vi "ZoomAndCenterImage.vi"(8 "error in (no error)":errorcluster, 10 "image data":T1, 11 "Picture Ref":refnum<vi>) -> (0 "error out":errorcluster)   [LabVIEW 2015]
uses:
  <vilib>/picture/picture.llb/imagedata.ctl
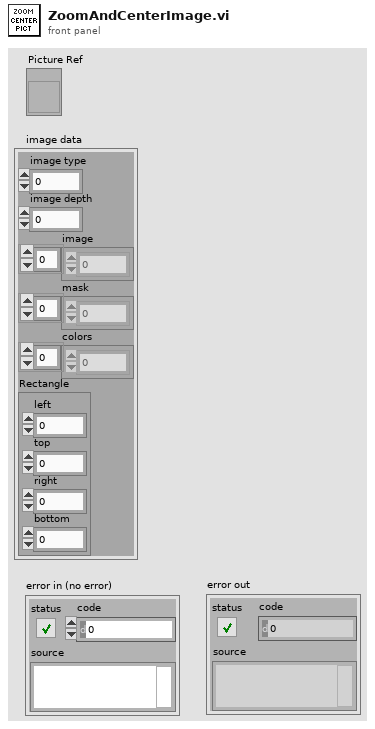
[diagram p1: front panel]
types:
  T1 = typedef "imagedata.ctl" = cluster{"image type":i32, "image depth":i32, "image":u8[], "mask":u8[], "colors":u32[], "Rectangle":cluster{"left":i16, "top":i16, "right":i16, "bottom":i16}}
  T2 = cluster{"left":i16, "top":i16, "right":i16, "bottom":i16}
  T3 = typedef "LVBoundsTypeDef.ctl" = cluster{"Width":u32, "Height":u32}
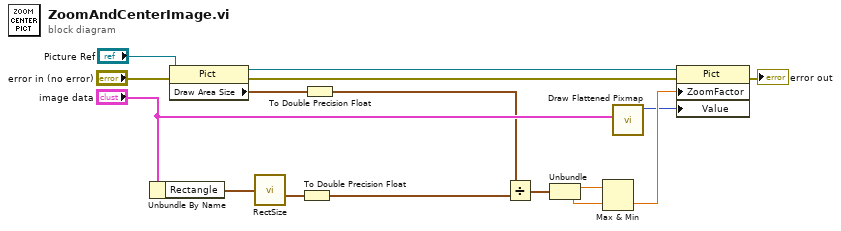
[diagram p0: block diagram]
diagram:
  n1 = Unbundle By Name("image data") -> ("Rectangle"=w16:T2)
  n2 = property class="Pict"(reference="Picture Ref", error in="error in (no error)") -> (reference out=w12:refnum<vi>, error out=w13:errorcluster, "Draw Area Size"=w10:T3)
  n3 = call <vilib>:"RectSize.vi"("rect"=w16) -> ("point"=w1:cluster{"x":i16, "y":i16})
  n4 = To Double Precision Float(number=w1) -> (double precision float=w3:cluster{"x":dbl, "y":dbl})
  n5 = To Double Precision Float(number=w10) -> (double precision float=w4:cluster{"Width":dbl, "Height":dbl})
  n6 = Divide(x=w4, y=w3) -> (x/y=w2:cluster{dbl, dbl})
  n7 = Unbundle(w2) -> (w9:dbl, w8:dbl)
  n8 = Max & Min(x=w9, y=w8) -> (min(x,y)=w7:dbl)  [unwired: 1 out]
  n9 = call <vilib>:"Draw Flattened Pixmap.vi"("image data"="image data") -> ("new picture"=w5:picture)  [unwired: 8 in]
  n10 = property class="Pict"(reference=w12, error in=w13, "ZoomFactor"=w7, "Value"=w5) -> (error out=→"error out":errorcluster)  [unwired: 1 out]
